vi "Knock Cylinder 1.0 In Place Input Write Structure.vi"(5 "Device Inputs":dbl[](array[numeric]), 7 "Last Device Inputs":dbl[](array[numeric]), 8 "error in (no error)":errorcluster, 9 "FPGA ref in":T1, 11 "1.0.0 Knock Cylinder in":T2) -> (0 "error out":errorcluster, 1 "FPGA ref out":T1, 3 "1.0.0 Knock Cylinder out":T2)   [LabVIEW 2019, in "Engine Simulation Toolkit Engine.lvlib"]
uses:
  Engine Simulation Toolkit Engine.lvlib
  Shared/1.0 Knock Cylinder Engine Data.ctl
  Shared/1.0 Knock Cylinder FIFO Idxs.ctl
  Knock Cylinder 1.0 Input Ref.ctl
  Shared/Probability % to compare.vi
  Shared/Angle in degrees to u16.vi
  Knock Cylinder 1.0 FPGA Inputs Write Node.vi
  Shared/Engine Simulation Toolkit Shared.lvlib
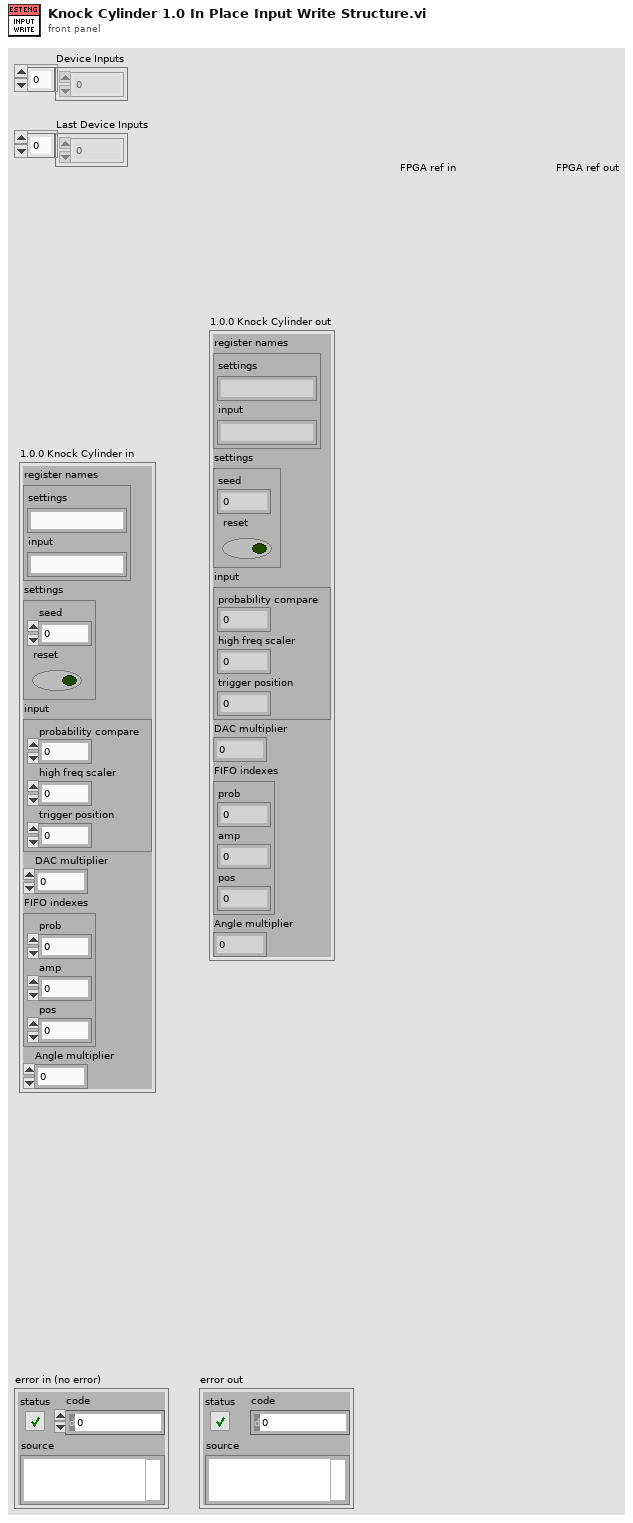
[diagram p1: front panel]
types:
  T1 = typedef "Engine Simulation Toolkit Engine.lvlib/Knock Cylinder 1.0 Input Ref.ctl" = refnum<k20>
  T2 = typedef "Engine Simulation Toolkit Shared.lvlib/1.0 Knock Cylinder Engine Data.ctl" = cluster{"register names":cluster{"settings":string, "input":string}, "settings":cluster{"seed":u16, "reset":bool}, "input":cluster{"probability compare":u16, "high freq scaler":fxp<+,10,0>, "trigger position":u16}, "DAC multiplier":dbl, "FIFO indexes":T3, "Angle multiplier":dbl}
  T3 = typedef "Engine Simulation Toolkit Shared.lvlib/1.0 Knock Cylinder FIFO Idxs.ctl" = cluster{"prob":i32, "amp":i32, "pos":i32}
  T4 = cluster{"probability compare":u16, "high freq scaler":fxp<+,10,0>, "trigger position":u16}
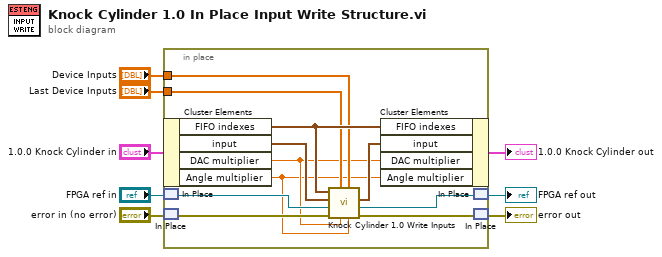
[diagram p0: block diagram]
diagram:
  n1 = in-place {
    in-place-border: "Last Device Inputs" -> [w14]
    in-place-border: "Device Inputs" -> [w13]
    n2 = in-place-cluster #1("1.0.0 Knock Cylinder in") -> ("FIFO indexes"=w16:T3, "input"=w17:T4, "DAC multiplier"=w10:dbl, "Angle multiplier"=w9:dbl)
    n3 = in-place-match #2("FPGA ref in") -> (w12:T1)
    n4 = in-place-match #3("error in (no error)") -> (w19:errorcluster)
    n5 = call "Knock Cylinder 1.0 Write Inputs.vi"("Angle multiplier"=w9, "Device inputs"=w13, "DAC multiplier"=w10, "Last Device inputs"=w14, "error in (no error)"=w19, "input reference in"=w12, "input in"=w17, "FIFO indexes.inputs"=w16) -> ("error out"=w18:errorcluster, "input reference out"=w11:T1, "input out"=w15:T4)  [unwired: 1 in]
    n6 = in-place-cluster #1("FIFO indexes"=w16, "input"=w15, "DAC multiplier"=w10, "Angle multiplier"=w9) -> (→"1.0.0 Knock Cylinder out":T2)
    n7 = in-place-match #2(w11) -> (→"FPGA ref out":T1)
    n8 = in-place-match #3(w18) -> (→"error out":errorcluster)
  }
